vi "Atto DRY Interface get Action Message.vi"(8 "error in (no error)":errorcluster, 10 "len":i32, 11 "ActionMessage":string) -> (0 "error out":errorcluster, 2 "function return":i32, 3 "ActionMessage out":string)   [LabVIEW 2016, in "attoDRYLib.lvlib"]
doc: "int32_t __cdecl AttoDRY_Interface_getActionMessage(char ActionMessage[], \n int32_t len);"
uses:
  <userlib>/attoDRYLib/attoDRYLib.lvlib
  <userlib>/attoDRYLib/attoDRYLib.dll
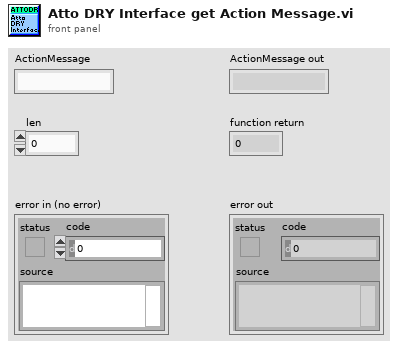
[diagram p1: front panel]
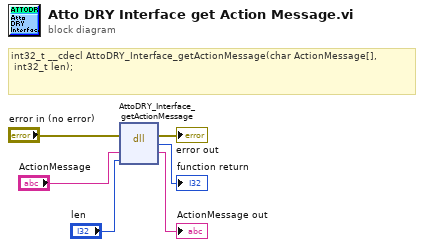
[diagram p0: block diagram]
diagram:
  # "int32_t __cdecl AttoDRY_Interface_getActionMessage(char ActionMessage[], \n\tint32_t len);"
  n1 = dll-call lib="C:/Program Files (x86)/National Instruments/LabVIEW 2016/user.lib/attoDRYLib/attoDRYLib.*" fn="AttoDRY_Interface_getActionMessage"(error in="error in (no error)", "ActionMessage"="ActionMessage", "len"="len") -> (error out=→"error out":errorcluster, →"function return":i32, "ActionMessage"=→"ActionMessage out":string)  [unwired: 3 in, 1 out]
